vi "Write data.vi"(8 "error in":errorcluster, 9 "starting address":u16, 10 "register value to write":u16, 11 "Modbus master in":refnum<class "Modbus Master.lvclass">) -> (0 "error out":errorcluster, 3 "Modbus master out":refnum<class "Modbus Master.lvclass">)   [LabVIEW 2023, in "RS485.lvlib"]
uses:
  RS485.lvlib
  <vilib>/NI/Modbus Library/API/Master/Modbus Master.lvclass
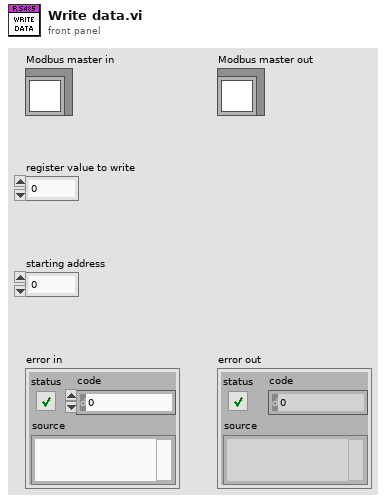
[diagram p1: front panel]
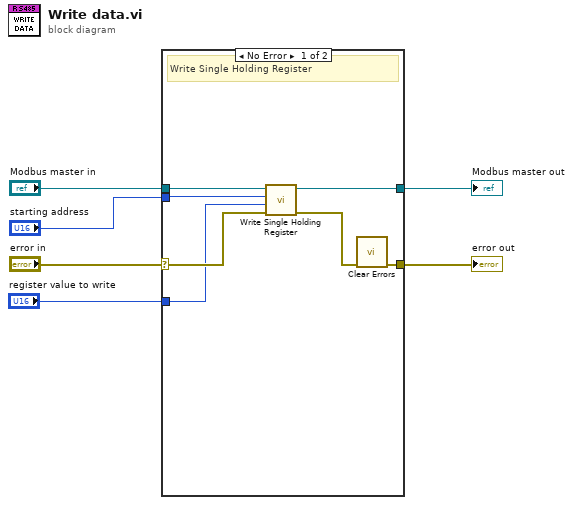
[diagram p0: block diagram]
diagram:
  n1 = case shown="No Error" "error in" {
    selector: "error in" -> [w11 w14]
    tunnel: "Modbus master in" -> [w13 w15]
    tunnel: [w12 w15] -> w3
    tunnel: [w7 w14] -> w2
    tunnel: "starting address" -> [w9 _]
    tunnel: "register value to write" -> [w8 _]
    frame No Error {
      # "Write Single Holding Register"
      n2 = call-dynamic "Write Single Holding Register.vi"("error in"=w11, "register to write"=w8, "address"=w9, "Modbus master in"=w13) -> ("error out"=w10:errorcluster, "Modbus master out"=w12:refnum<class "Modbus Master.lvclass">)  [unwired: 6 in]
      n3 = call <vilib>:"Clear Errors.vi"("error in (no error)"=w10) -> ("error out"=w7:errorcluster)  [unwired: 5 in, 1 out]
    }
    frame Error {
      # "Error in Initialization"
    }
  }
  "Modbus master out" <- w3
  "error out" <- w2
